vi "Stop Aquisition.vi"(8 "error in (no error)":errorcluster, 11 "HRF_Device":refnum<class "HRF_Device.lvclass">) -> (0 "error out":errorcluster, 3 "HRF_Device":refnum<class "HRF_Device.lvclass">)   [LabVIEW 2020, in "HRF_Device.lvclass"]
uses:
  HRF_Device.lvclass
  HRF_Device.lvclass/HRF_Device.ctl
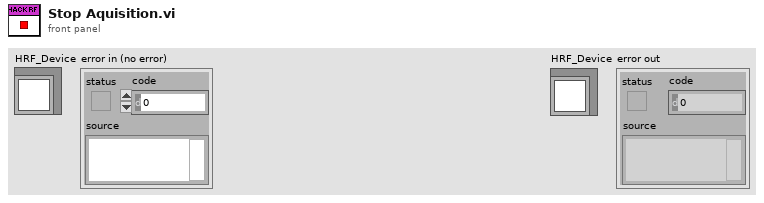
[diagram p1: front panel]
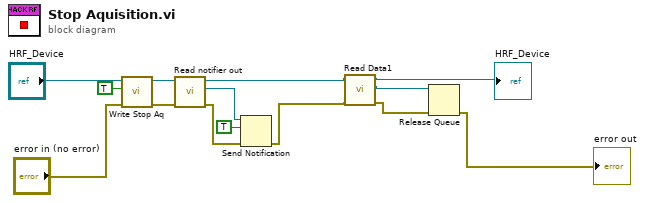
[diagram p0: block diagram]
diagram:
  n1 = call "Write Stop Aq.vi"("error in (no error)"="error in (no error)", "Stop Aq"=TRUE, "HRF_Device in"="HRF_Device") -> ("error out"=w10:errorcluster, "HRF_Device out"=w11:refnum<class "HRF_Device.lvclass">)  [unwired: 7 in]
  n2 = call "Read notifier out.vi"("error in (no error)"=w10, "HRF_Device in"=w11) -> ("error out"=w8:errorcluster, "notifier out"=w9:refnum<notifier>, "HRF_Device out"=w6:refnum<class "HRF_Device.lvclass">)  [unwired: 7 in]
  n3 = Send Notification(notification=TRUE, notifier=w9, error in (no error)=w8) -> (error out=w3:errorcluster)  [unwired: 1 out]
  n4 = call "Read Data1.vi"("error in (no error)"=w3, "HRF_Device in"=w6) -> ("error out"=w2:errorcluster, "Data"=w4:refnum<queue>, "HRF_Device out"=→"HRF_Device":refnum<class "HRF_Device.lvclass">)  [unwired: 7 in]
  n5 = Release Queue(queue=w4, error in (no error)=w2) -> (error out=→"error out":errorcluster)  [unwired: 1 in, 2 out]
